vi "GetLocalConfiguration.vi"() -> (1 "Configuration File":path=path "C:/Users/itk/Documents/itk-strip-sensor-qc/QCtests/general_VIs/LocalConfig/QCconfig.txt")   [LabVIEW 2018]
uses:
  globals/QC_RunInformation.vi
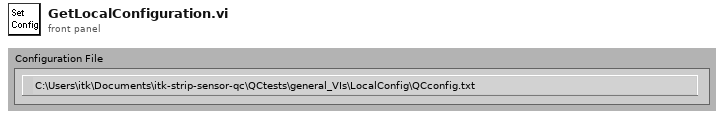
[diagram p1: front panel]
types:
  T1 = cluster{"Institute":string, "Manufacturers":string[], "Devices":string[], "Serialnumbers Lookup DB":string, "Data directory":string, "Backup & screenshot directory":string, "List of known users":string[]}
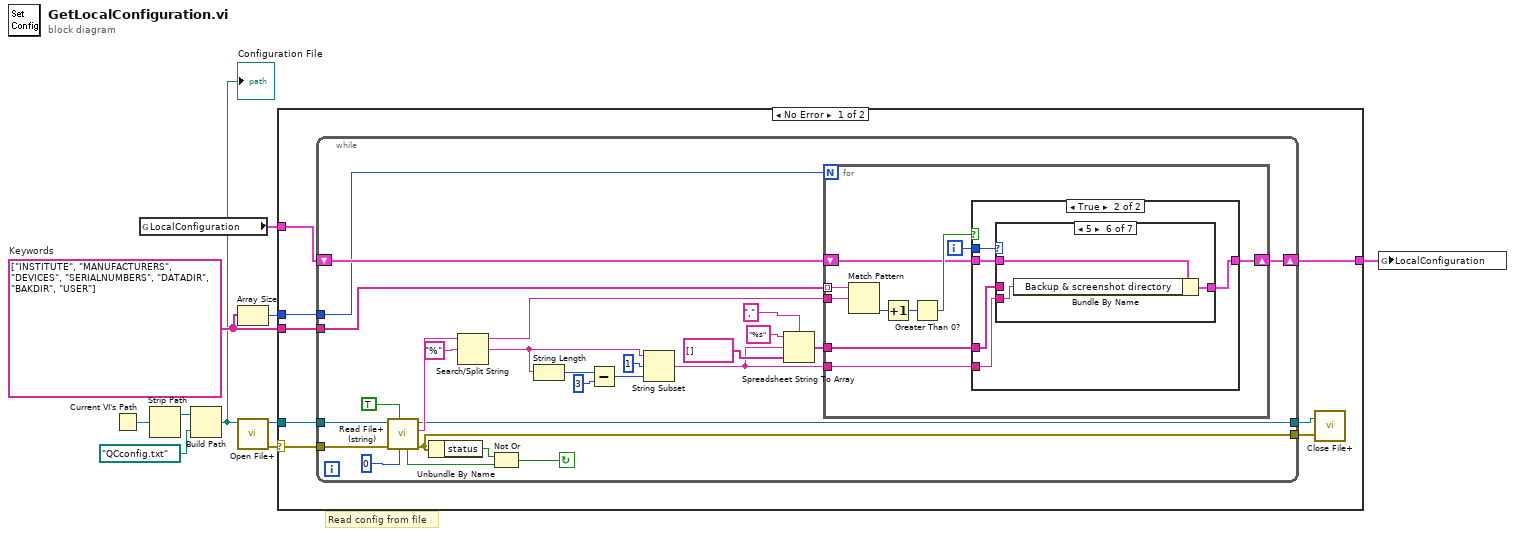
[diagram p0: block diagram]
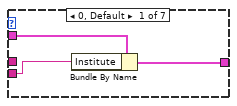
[diagram p3: hidden frame]
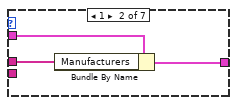
[diagram p4: hidden frame]
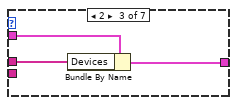
[diagram p5: hidden frame]
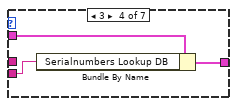
[diagram p6: hidden frame]
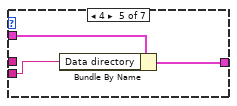
[diagram p7: hidden frame]
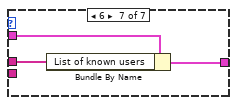
[diagram p8: hidden frame]
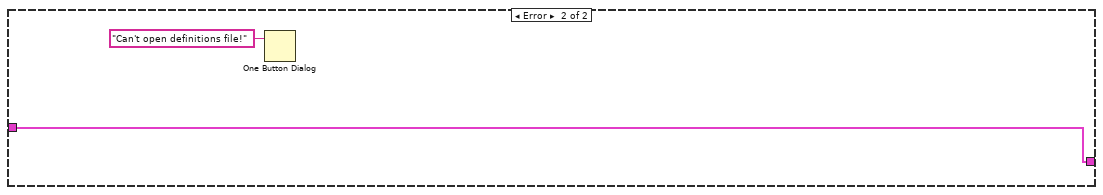
[diagram p9: hidden frame]
diagram:
  w10 = string[] ["INSTITUTE", "MANUFACTURERS", "DEVICES", "SERIALNUMBERS", "DATADIR", "BAKDIR", "USER"]  # Keywords
  # "Read config from file"
  n1 = Current VI's Path() -> (path=w3:path)
  n2 = global read "QC_RunInformation.vi" "LocalConfiguration"() -> (w8:T1)
  n3 = Strip Path(path=w3) -> (stripped path=w2:path)  [unwired: 1 out]
  n4 = Build Path(base path=w2, name or relative path=path "QCconfig.txt") -> (appended path=w1:path)
  "Configuration File" <- w1
  n5 = Array Size(array=w10) -> (size(s)=w9:i32)
  n6 = call <vilib>:"Open File+.vi"("file path (\" \")"=w1) -> ("error out"=w4:errorcluster, "refnum"=w5:refnum<file>)  [unwired: 7 in, 2 out]
  n7 = case shown="No Error" w4 {
    selector: w4 -> [w11 _]
    tunnel: w5 -> [w18 _]
    tunnel: w10 -> [w17 _]
    tunnel: w9 -> [w16 _]
    tunnel: w8 -> [w15 w82]
    tunnel: [w14 w82] -> w6
    frame No Error {
      n8 = while {
        shift-left: w15 -> [w22]
        shift-right: [w20] -> w14
        tunnel: w16 -> [w19]
        tunnel: w17 -> [w26]
        tunnel: [w30] -> w12
        tunnel: w11 -> [w31]
        tunnel: [w32] -> w13
        tunnel: w18 -> [w38]
        stop <- w34 continue-if-true
        n9 = call <vilib>:"Read File+ (string).vi"("count"=0, "line mode (characters:F)"=TRUE, "error in (no error)"=w31, "refnum"=w38) -> ("error out"=w30:errorcluster, "string"=w33:string, "dup refnum"=w32:refnum<file>, "EOF?"=w36:bool)  [unwired: 3 in, 1 out]
        n10 = Unbundle By Name(w30) -> ("status"=w35:bool)
        n11 = Search/Split String(string=w33, search string/char (-)="%" ("search char (-)")) -> (substring before match=w25:string, match + rest of string=w40:string)  [unwired: 1 in, 1 out]
        n12 = Not Or(1:w36, 2:w35) -> (0:w34:bool)
        n13 = String Length(string=w40) -> (length=w23:i32)
        n14 = Subtract(x=w23, y=3) -> (x-y=w27:i32)
        n15 = String Subset(string=w40, offset (0)=1, length (rest)=w27) -> (substring=w21:string)
        n16 = Spreadsheet String To Array(delimiter (Tab)=",", format string="%s", spreadsheet string=w21, array type (2D Dbl)=string[] []) -> (array=w24:string[])
        n17 = for {
          N: w19 -> [_]
          tunnel: w26 -> [w52] mode=indexing
          tunnel: w25 -> [w46]
          tunnel: w24 -> [w49]
          shift-right: [w47] -> w20
          shift-left: w22 -> [w48]
          tunnel: w21 -> [w45]
          i -> [w50]
          n18 = Match Pattern(string=w52, regular expression=w46) -> (offset past match=w53:i32)  [unwired: 1 in, 3 out]
          n19 = Increment(x=w53) -> (x+1=w54:i32)
          n20 = Greater Than 0?(x=w54) -> (x > 0?=w51:bool)
          n21 = case shown="True" w51 {
            tunnel: w50 -> [_ w60]
            tunnel: w49 -> [_ w59]
            tunnel: w45 -> [_ w58]
            tunnel: w48 -> [w55 w57]
            tunnel: [w55 w56] -> w47
            frame False {
            }
            frame True {
              n22 = case shown="5" w60 {
                tunnel: w59 -> [_ w65 w68 _ _ _ w79]
                tunnel: w58 -> [w61 _ _ w70 w73 w76 _]
                tunnel: w57 -> [w63 w66 w69 w72 w75 w78 w81]
                tunnel: [w62 w64 w67 w71 w74 w77 w80] -> w56
                frame 0, Default {
                  n23 = Bundle By Name(cluster=w63, "Institute"=w61) -> (w62:T1)
                }
                frame 1 {
                  n24 = Bundle By Name(cluster=w66, "Manufacturers"=w65) -> (w64:T1)
                }
                frame 2 {
                  n25 = Bundle By Name(cluster=w69, "Devices"=w68) -> (w67:T1)
                }
                frame 3 {
                  n26 = Bundle By Name(cluster=w72, "Serialnumbers Lookup DB"=w70) -> (w71:T1)
                }
                frame 4 {
                  n27 = Bundle By Name(cluster=w75, "Data directory"=w73) -> (w74:T1)
                }
                frame 5 {
                  n28 = Bundle By Name(cluster=w78, "Backup & screenshot directory"=w76) -> (w77:T1)
                }
                frame 6 {
                  n29 = Bundle By Name(cluster=w81, "List of known users"=w79) -> (w80:T1)
                }
              }
            }
          }
        }
      }
      n30 = call <vilib>:"Close File+.vi"("error in (no error)"=w12, "refnum"=w13) -> ()  [unwired: 3 in, 3 out]
    }
    frame Error {
      n31 = One Button Dialog(message="Can't open definitions file!") -> ()  [unwired: 1 in, 1 out]
    }
  }
  n32 = global write "QC_RunInformation.vi" "LocalConfiguration"(w6) -> ()
